vi "Write Index.vi"(8 "error in":errorcluster, 10 "index":i32, 11 "channel in":refnum<class "Channel.lvclass">) -> (0 "error out":errorcluster, 3 "channel out":refnum<class "Channel.lvclass">)   [LabVIEW 2017, in "Scan Engine Scripting.lvlib" / "Channel.lvclass"]
doc: "Writes the index to the private data of the channel."
uses:
  Channel.lvclass
  Channel.lvclass/Channel.ctl
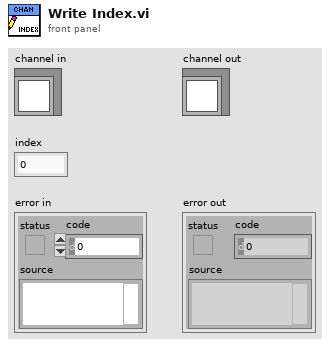
[diagram p1: front panel]
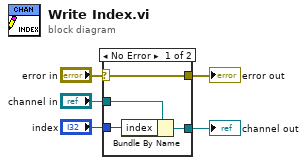
[diagram p0: block diagram]
diagram:
  n1 = case shown="No Error" "error in" {
    selector: "error in" -> [w9 w10]
    tunnel: [w9 w10] -> w4
    tunnel: [w7 w11] -> w2
    tunnel: "channel in" -> [w8 w11]
    tunnel: "index" -> [w6 _]
    frame No Error {
      n2 = Bundle By Name(cluster=w8, "index"=w6) -> (w7:refnum<class "Channel.lvclass">)
    }
    frame Error {
    }
  }
  "error out" <- w4
  "channel out" <- w2
